vi "Lorentz Fit Test.vi"() -> ()   [LabVIEW 2016]
uses:
  LabActor/Post-Processors/Line Detector/Resonance Detector Configuration.ctl
panel:
  out "XY Graph":cluster{"X":dbl[], "Array":dbl[]}[](graph)
  out "best fit parameters":dbl[](array[numeric]) format="%#_9g"
  in  "Guess":dbl[](array[numeric])=[932285.0, 10.0, 0.005, 1.0, 0.002, 0.001] format="%#_9p"
  in  "File":path=path "C:/Data/URu2Si2/9.42740K_480_2000_0.55218V_Jul09-2013__00-01-46_001_070913.tdms"
  in  "Line Detector Configuration":T1={"Peak width guess"=100.0, "Background removal"=enum."NONE", "Smoothing"=enum."NONE", "Smooth window"=100.0, "Relative threshold"=0.0, "Finder algorithm"=enum."Basic", "Bgd window"=100.0, "Spectrum recorder module name"="Spectrum Recorder", "Fit window"=100.0, "Initial fit guess"=enum."Last fit", "...with header "="", "Follow\npeaks"=FALSE, "Re-sample"=nan, "rusin\n.dat"=enum."NONE"} {"Re-sample" format="%#_6pHz"; "Fit window" format="%#_6pHz"; "Bgd window" format="%#_6pHz"; "Smooth window" format="%#_6pHz"; "Peak width guess" format="%#_6pHz"}
  # "Peak finder config"
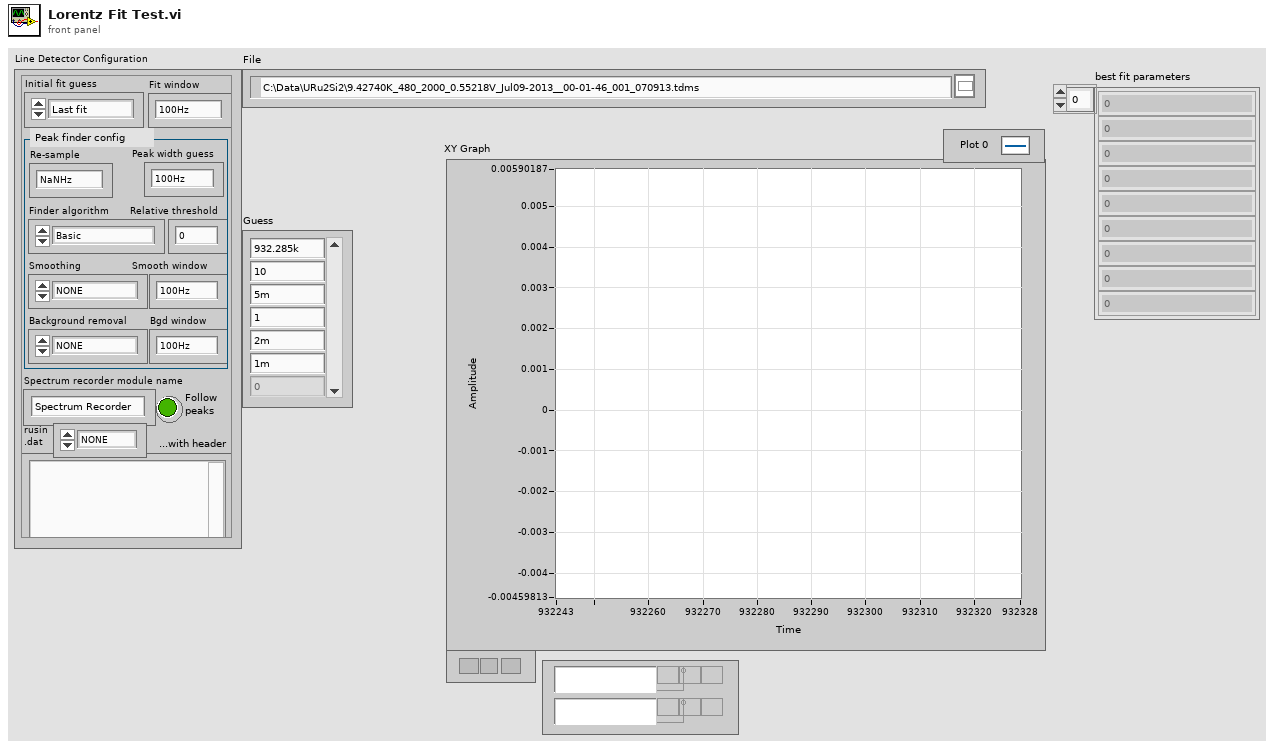
[diagram p1: front panel]
types:
  T1 = typedef "Line Detector Configuration.ctl" = cluster{"Peak width guess":dbl, "Background removal":enum16{"NONE", "High-pass", "Detrend"}, "Smoothing":enum16{"NONE", "Low-pass", "Denoise"}, "Smooth window":dbl, "Relative threshold":dbl, "Finder algorithm":enum16{"Basic", "Wavelet", "Wavelet+detrend"}, "Bgd window":dbl, "Spectrum recorder module name":string, "Fit window":dbl, "Initial fit guess":enum16{"Peak finder", "Last fit"}, "...with header ":string, "Follow\npeaks":bool, "Re-sample":dbl, "rusin\n.dat":enum16{"NONE", "DINES/cm2", "GPa"}}
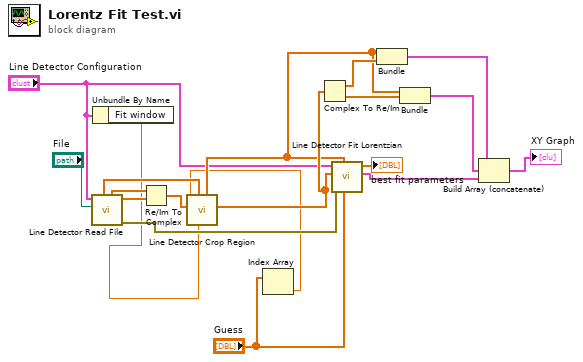
[diagram p0: block diagram]
diagram:
  n1 = call "Line Detector Read File.vi"("File"="File", "Line Detector Configuration"="Line Detector Configuration") -> ("error out"=w14:errorcluster, "Signal Y"=w17:dbl[], "Signal X"=w18:dbl[], "Frequency"=w15:dbl[])  [unwired: 2 in, 4 out]
  n2 = Unbundle By Name("Line Detector Configuration") -> ("Fit window"=w3:dbl)
  n3 = Re/Im To Complex(1:w17, 2:w18) -> (0:w16:cdb[])
  n4 = Index Array(array="Guess") -> (element=w1:dbl)  [unwired: 1 in]
  n5 = call "Line Detector Crop Region.vi"("Region width"=w3, "Frequency"=w15, "Signal"=w16, "Center frequency"=w1) -> ("Signal  out"=w8:cdb[], "Frequency out"=w5:dbl[])  [unwired: 4 in, 2 out]
  n6 = Complex To Re/Im(x + iy=w8) -> (x=w7:dbl[], y=w6:dbl[])
  n7 = call "Line Detector Fit Lorentzian.vi"("Guess"="Guess", "Frequency"=w5, "Error In"=w14, "Signal"=w8, "Line Detector Configuration"="Line Detector Configuration") -> ("Plot"=w12:cluster{"X":dbl[], "Array":dbl[]}[], "best fit parameters"=→"best fit parameters":dbl[])  [unwired: 4 in, 1 out]
  n8 = Bundle("Frequency out"=w5, w7) -> (w9:cluster{"Frequency out":dbl[], dbl[]})  [unwired: 1 in]
  n9 = Bundle("Frequency out"=w5, w6) -> (w10:cluster{"Frequency out":dbl[], dbl[]})  [unwired: 1 in]
  n10 = Build Array (concatenate)(w9, w10, w12) -> (→"XY Graph":cluster{"X":dbl[], "Array":dbl[]}[])
